vi "NodeConfiguration_Create.vi"(0 "reference in":refnum<class "NodeConfiguration.lvclass">, 1 "ConfigFile":path, 5 "error in (no error)":errorcluster) -> (14 "reference out":refnum<class "NodeConfiguration.lvclass">, 19 "error out":errorcluster)   [LabVIEW 2014, in "NodeConfiguration.lvclass"]
uses:
  NodeConfiguration.lvclass
  Config.ctl
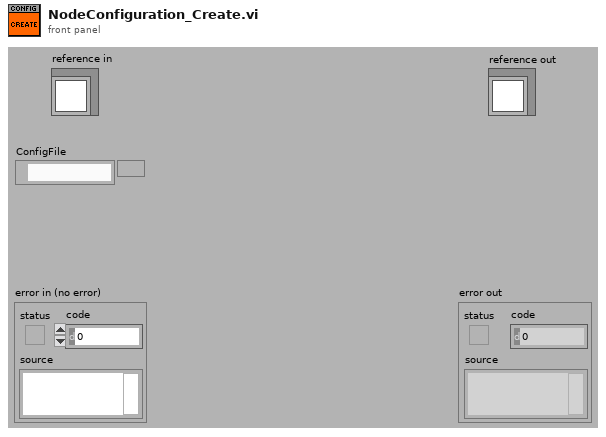
[diagram p1: front panel]
types:
  T1 = typedef "NodeConfiguration.lvclass/Config.ctl" = cluster{"NodeName":string, "TemperatureOffset":dbl, "RH Offset":dbl}
  T2 = typedef "NodeConfiguration.lvclass/ObjectAttributes.ctl" = cluster{"Config":T1, "ConfigFile":path}
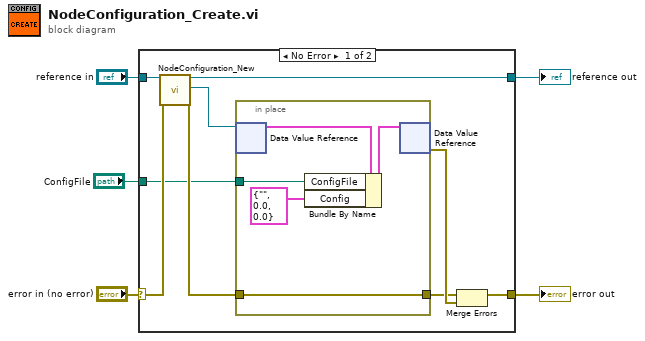
[diagram p0: block diagram]
diagram:
  n1 = case shown="No Error" "error in (no error)" {
    selector: "error in (no error)" -> [w13 w21]
    tunnel: [w10 w21] -> w4
    tunnel: "reference in" -> [w14 w20]
    tunnel: [w12 w20] -> w2
    tunnel: "ConfigFile" -> [w6 _]
    frame No Error {
      n2 = call "NodeConfiguration_New.vi"("reference in"=w14, "error in (no error)"=w13) -> ("reference out"=w12:refnum<class "NodeConfiguration.lvclass">, "DVRRefOut"=w9:refnum<data-value>, "error out"=w8:errorcluster)  [unwired: 14 in, 1 out]
      n3 = in-place {
        in-place-border: w8 -> [w17]
        in-place-border: [w17] -> w7
        in-place-border: w6 -> [w16]
        n4 = in-place-dvr #1(w9) -> (w18:T2)  [unwired: 1 out]
        n5 = Bundle By Name(cluster=w18, "ConfigFile"=w16, "Config"=T1 {"NodeName"="", "TemperatureOffset"=0.0, "RH Offset"=0.0}) -> (w19:T2)
        n6 = in-place-dvr #1(w19) -> (w11:errorcluster)  [unwired: 1 out]
      }
      n7 = Merge Errors(w7, w11) -> (w10:errorcluster)
    }
    frame Error {
      # "VI-TechBaseTemplate_Simple_6x8x6"
    }
  }
  "error out" <- w4
  "reference out" <- w2
